vi "power.vi"   [LabVIEW 2023, in "LabGRAD.lvlib" / "Value.lvclass"]
uses:
  Value.lvclass
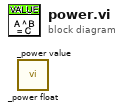
[diagram p0: block diagram]
diagram:
  n1 = call "_power float.vi"() -> ()  [unwired: 9 in, 3 out]
  n2 = call "_power value.vi"() -> ()  [unwired: 9 in, 3 out]
